vi "Get SMO Database Paths.vi"(5 "getAll Cluster":variant, 7 "Paths":string="llab_038:d000(TEST_TABLE--Temperature(Kelvin))\nllab_038:d002(TEST_TABLE--voltage 2(volts))\nllab_038:b000(TEST_TABLE--ON?())\nllab_038:v001(TEST_TABLE--sample())", 8 "error in (no error)":errorcluster, 11 "Instrument.Framework-Template in":refnum<class "Instrument.Framework-Template.lvclass">) -> (0 "error out":errorcluster, 2 "Paths":string, 3 "Instrument.Framework-Template out":refnum<class "Instrument.Framework-Template.lvclass">)   [LabVIEW 2019, in "Instrument.Framework-Template.lvclass"]
uses:
  Instrument.Framework-Template.lvclass
  Typedefs/Instrument.Framework-Template.getAll--Cluster.ctl
  Framework/Instrument Types/SCPI/Instrument.SCPI.lvclass
  <userlib>/LevyLab/LV-Data/LV-Data.PG/LV-Data.PGSQL.lvclass
  <userlib>/LevyLab/LV-Data/LV-Data.PG/API/Write Variable (one-row).vi
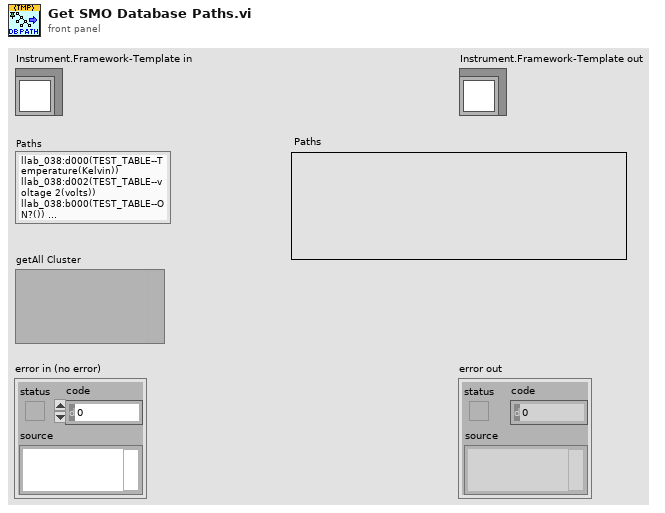
[diagram p1: front panel]
types:
  T1 = typedef "Instrument.Framework-Template.lvclass/Instrument.Framework-Template.getAll--Cluster.ctl" = cluster{"Levy 1":dbl, "Logger SMO":dbl, "SMO Boolean":bool, "SMO String":string}
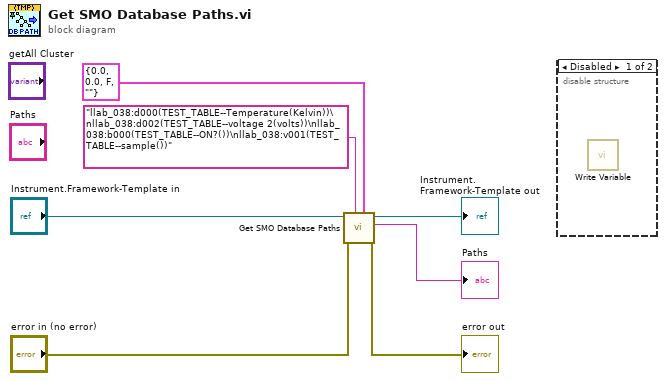
[diagram p0: block diagram]
diagram:
  n1 = call-parent "Get SMO Database Paths.vi"("getAll Cluster"=T1 {"Levy 1"=0.0, "Logger SMO"=0.0, "SMO Boolean"=FALSE, "SMO String"=""} ("getAll"), "Default Paths"="llab_038:d000(TEST_TABLE--Temperature(Kelvin))\nllab_038:d002(TEST_TABLE--voltage 2(volts))\nllab_038:b000(TEST_TABLE--ON?())\nllab_038:v001(TEST_TABLE--sample())" ("Paths"), "error in (no error)"="error in (no error)", "Instrument in"="Instrument.Framework-Template in") -> ("error out"=→"error out":errorcluster, "Paths"=→"Paths":string, "Instrument out"=→"Instrument.Framework-Template out":refnum<class "Instrument.Framework-Template.lvclass">)  [unwired: 5 in]
  n2 = disable-structure shown="Disabled" {
    frame Disabled {
      n3 = call-poly <userlib>:"Write Variable.vi"() -> ()  [unwired: 8 in, 4 out]
    }
    frame Enabled {
    }
  }
